vi "kinectRead [DepthFrame].vi"(8 "error in (no error)":errorcluster, 11 "KinectSensor References in":T1) -> (0 "error out":errorcluster, 2 "frameData":u8[](array[numeric]), 3 "KinectSensor References out":T1)   [LabVIEW 2014]
uses:
  Microsoft.Kinect
  controls/KinectSensor References.ctl
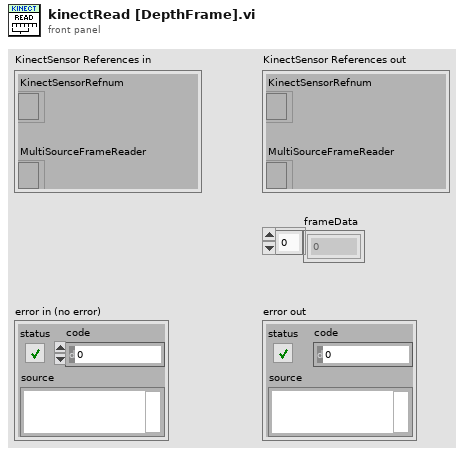
[diagram p1: front panel]
types:
  T1 = typedef "KinectSensor References.ctl" = cluster{"KinectSensorRefnum":refnum<k24>, "MultiSourceFrameReader":refnum<k24>}
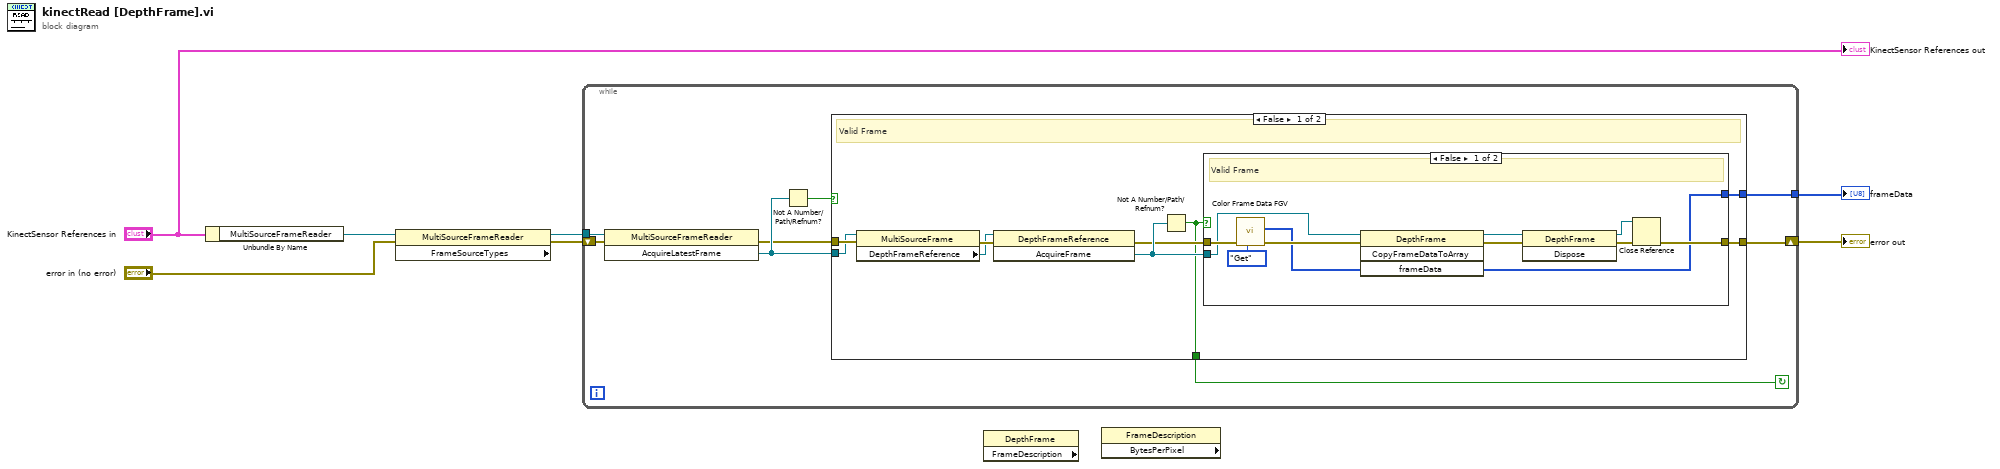
[diagram p0: block diagram]
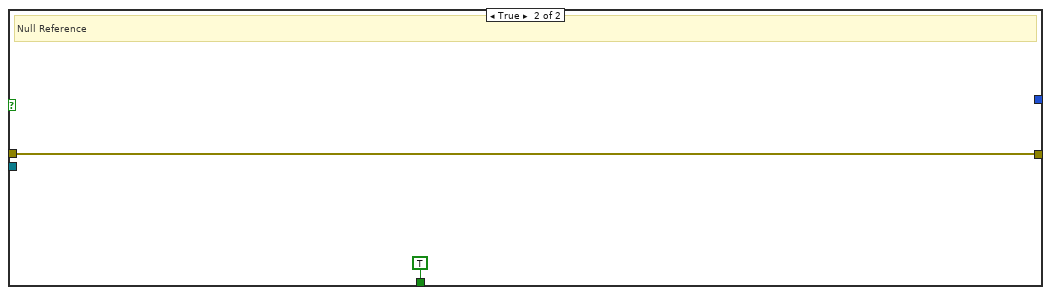
[diagram p3: hidden frame]
diagram:
  n1 = Unbundle By Name("KinectSensor References in") -> ("MultiSourceFrameReader"=w5:refnum<k24>)
  n2 = property class="MultiSourceFrameReader" props=["FrameSourceTypes"](reference=w5, error in="error in (no error)") -> (reference out=w7:refnum<k24>, error out=w6:errorcluster)  [unwired: 1 out]
  n3 = while {
    tunnel: w7 -> [w15]
    shift-right: [w10] -> w2
    shift-left: w6 -> [w14]
    tunnel: [w8] -> w1
    stop <- w9 continue-if-true
    n4 = invoke class="MultiSourceFrameReader" method="AcquireLatestFrame"(reference=w15, error in=w14) -> (error out=w12:errorcluster, "AcquireLatestFrame"=w13:refnum<k24>)  [unwired: 1 in, 1 out]
    n5 = Not A Number/Path/Refnum?(number/path/refnum=w13) -> (NaN/Path/Refnum?=w11:bool)
    n6 = case shown="False" w11 {
      tunnel: w12 -> [w21 w37]
      tunnel: w13 -> [w18 _]
      tunnel: [w20 w37] -> w10
      tunnel: [w19 TRUE] -> w9
      tunnel: [w16 _] -> w8
      frame False {
        # "Valid Frame"
        n7 = property class="MultiSourceFrame"(reference=w18, error in=w21) -> (error out=w22:errorcluster, "DepthFrameReference"=w17:refnum<k24>)  [unwired: 1 out]
        n8 = invoke class="DepthFrameReference" method="AcquireFrame"(reference=w17, error in=w22) -> (error out=w23:errorcluster, "AcquireFrame"=w24:refnum<k24>)  [unwired: 1 in, 1 out]
        n9 = Not A Number/Path/Refnum?(number/path/refnum=w24) -> (NaN/Path/Refnum?=w19:bool)
        n10 = case shown="False" w19 {
          tunnel: w23 -> [w28 w36]
          tunnel: w24 -> [w27 _]
          tunnel: [w26 w36] -> w20
          tunnel: [w25 _] -> w16
          frame False {
            # "Valid Frame"
            n11 = call "Color Frame Data FGV.vi"("Command"=enum16{"Get", "Initialize"}."Get", "error in (no error)"=w28) -> ("error out"=w35:errorcluster, "Byte Array"=w30:u8[])  [unwired: 8 in]
            n12 = invoke class="DepthFrame" method="CopyFrameDataToArray"(reference=w27, error in=w35, "frameData"=w30) -> (reference out=w31:refnum<k24>, error out=w32:errorcluster, "frameData"=w25:u16[])  [unwired: 1 in, 1 out]
            n13 = invoke class="DepthFrame" method="Dispose"(reference=w31, error in=w32) -> (reference out=w34:refnum<k24>, error out=w33:errorcluster)  [unwired: 1 in, 1 out]
            n14 = Close Reference(reference=w34, error in (no error)=w33) -> (error out=w26:errorcluster)
          }
          frame True {
            # "Null Reference"
          }
        }
      }
      frame True {
        # "Null Reference"
      }
    }
  }
  "error out" <- w2
  "frameData" <- w1
  n15 = property class="DepthFrame" props=["FrameDescription"]() -> ()  [unwired: 2 in, 3 out]
  n16 = property class="FrameDescription" props=["BytesPerPixel"]() -> ()  [unwired: 2 in, 3 out]
  "KinectSensor References out" <- "KinectSensor References in"
